vi "New.vi"(6 "Delimiters":T1={"Close"="}}", "Open"="{{"}, 8 "Error In":errorcluster, 11 "Key":string) -> (0 "Error Out":errorcluster, 3 "Partial":refnum<class "Partial.lvclass">)   [LabVIEW 2018, in "Toolkit.lvlib" / "Nodes.lvlib" / "Partial.lvclass"]
doc: "Creates a new Partial node that represents a Mustache Partial tag in a parsed template."
uses:
  Partial.lvclass
  Type Definitions/Delimiters.ctl
  Partial.lvclass/Partial.ctl
  Toolkit.lvlib
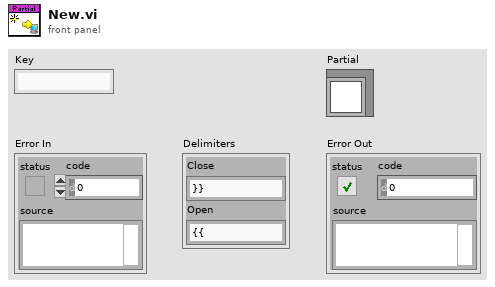
[diagram p1: front panel]
types:
  T1 = typedef "Toolkit.lvlib/Delimiters.ctl" = cluster{"Close":string, "Open":string}
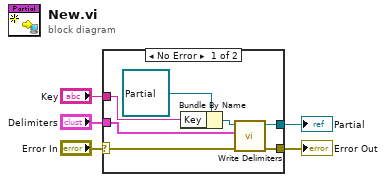
[diagram p0: block diagram]
diagram:
  n1 = case shown="No Error" "Error In" {
    selector: "Error In" -> [w9 w13]
    tunnel: "Key" -> [w10 _]
    tunnel: [w8 _] -> w3
    tunnel: [w7 w13] -> w2
    tunnel: "Delimiters" -> [w6 _]
    frame No Error {
      n2 = Bundle By Name(cluster=refnum<class "Partial.lvclass"> refnum ("Toolkit.lvlib:Nodes.lvlib:Partial.lvclass"), "Key"=w10) -> (w11:refnum<class "Partial.lvclass">)
      n3 = call-dynamic "Write Delimiters.vi"("Error In"=w9, "Delimiters"=w6, "Node In"=w11) -> ("Error Out"=w7:errorcluster, "Node Out"=w8:refnum<class "Partial.lvclass">)  [unwired: 7 in]
    }
    frame Error {
    }
  }
  "Partial" <- w3
  "Error Out" <- w2
